vi "RunCmd.vi"(9 "Cmd String":string, 11 "working directory":path=path "") -> (1 "OK":bool, 3 "Output":string)   [LabVIEW 2012]
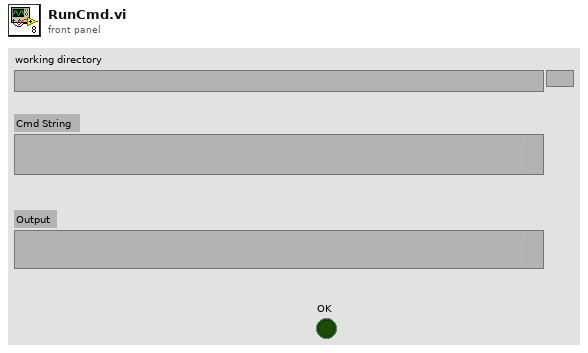
[diagram p1: front panel]
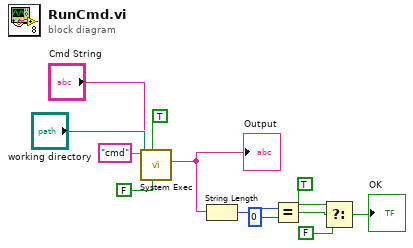
[diagram p0: block diagram]
diagram:
  n1 = call <vilib>:"System Exec.vi"("run minimized? (F)"=FALSE, "wait until completion? (T)"=TRUE, "working directory"="working directory", "standard input"="Cmd String", "command line"="cmd") -> ("standard error"=w7:string)  [unwired: 1 in, 5 out]
  "Output" <- w7
  n2 = String Length(string=w7) -> (length=w8:i32)
  n3 = Equal?(x=w8, y=0) -> (x = y?=w10:bool)
  n4 = Select(t=TRUE, s=w10, f=FALSE) -> (s? t:f=→"OK":bool)
